vi "Z_state.vi"(9 "Alarm":bool[](array[boolean])=[FALSE, FALSE], 10 "Z_In":T4={"Z_Source"=enum."hand", "Z_Set_State"=enum."initialization", "ZM_State"=enum."initialization"}, 11 "HE1_Z_state in":refnum<class "HE_Z_state.lvclass">) -> (3 "HE1_Z_state out":refnum<class "HE_Z_state.lvclass">)   [LabVIEW 2019, in "Heating.lvlib" / "HE_Z_state.lvclass"]
uses:
  HE_Z_state.lvclass
  D:/my_projects/projects/Algorithms/Labview/19/Sequence/State/State.lvclass
  ctl/Z_source.ctl
  ctl/Z_State.ctl
  ctl/ZM_State.ctl
  HE_Z_state.lvclass/HE_Z_state.ctl
  Sequence/State/State.lvclass
  Heating.lvlib
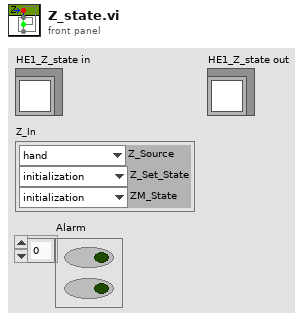
[diagram p1: front panel]
types:
  T1 = typedef "Heating.lvlib/Z_source.ctl" = enum8{"initialize", "local disabled", "local hand", "hand", "auto", "dist"}
  T2 = typedef "Heating.lvlib/Z_State.ctl" = enum8{"initialization", "alarm", "disabled", "not ready", "stop ready", "reserv", "switched off", "reserv2", "switched on", "check", "on min", "decrease out", "on", "increase out", "on max"}
  T3 = typedef "Heating.lvlib/ZM_State.ctl" = enum8{"initialization", "stop", "start_cmd", "contactor_on_cmd", "heating", "on", "stop_cmd", "power_down", "contactor_off_cmd", "cooling", "restart_delay"}
  T4 = cluster{"Z_Source":T1, "Z_Set_State":T2, "ZM_State":T3}
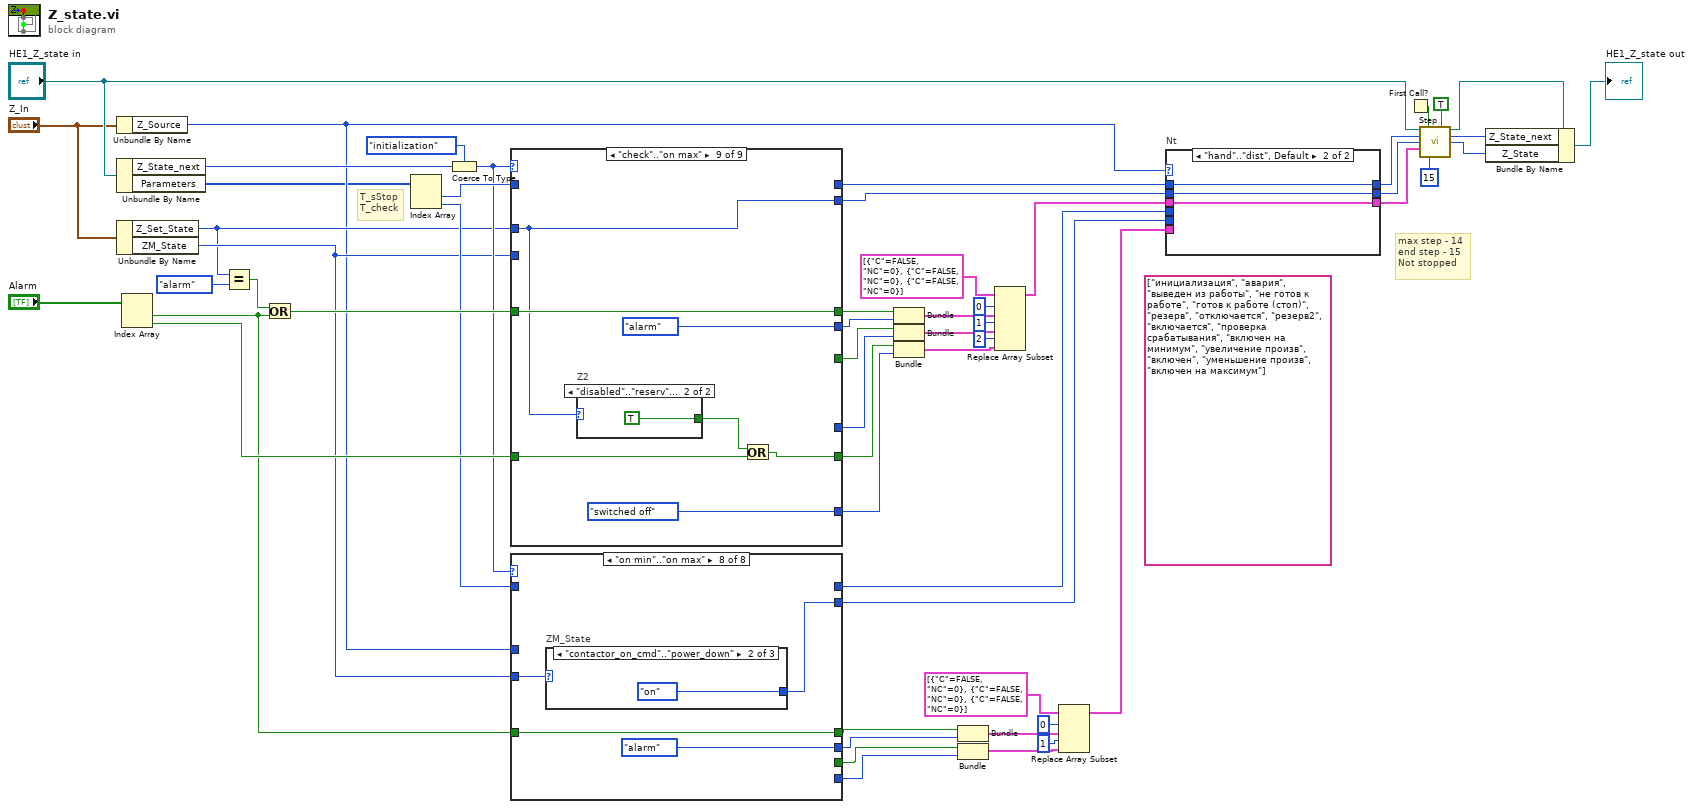
[diagram p0: block diagram]
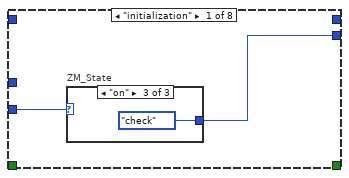
[diagram p2: hidden frame]
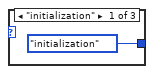
[diagram p3: hidden frame]
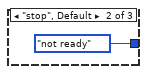
[diagram p4: hidden frame]
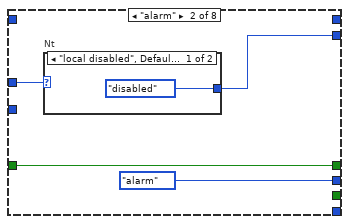
[diagram p5: hidden frame]
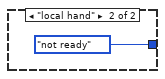
[diagram p6: hidden frame]
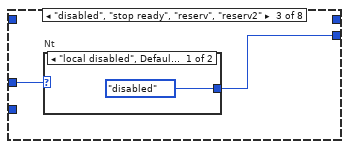
[diagram p7: hidden frame]
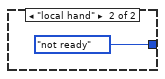
[diagram p8: hidden frame]
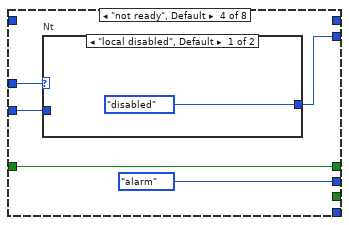
[diagram p9: hidden frame]
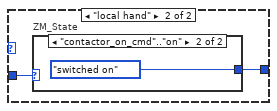
[diagram p10: hidden frame]
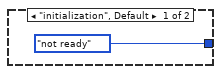
[diagram p11: hidden frame]
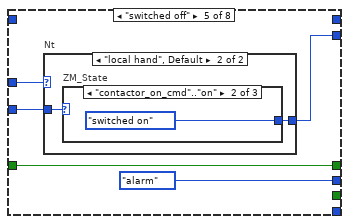
[diagram p12: hidden frame]
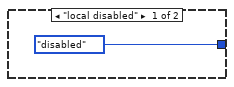
[diagram p13: hidden frame]
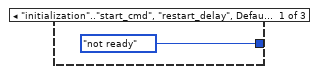
[diagram p14: hidden frame]
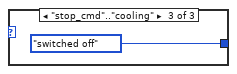
[diagram p15: hidden frame]
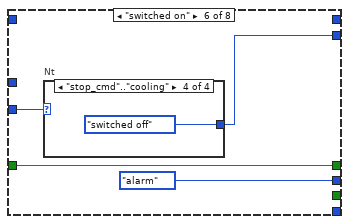
[diagram p16: hidden frame]
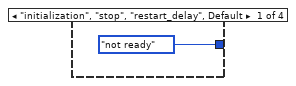
[diagram p17: hidden frame]
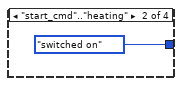
[diagram p18: hidden frame]
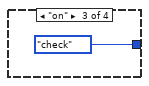
[diagram p19: hidden frame]
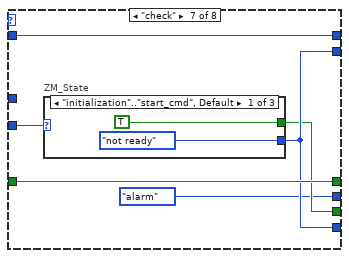
[diagram p20: hidden frame]
diagram:
  (unwired) string[] ["инициализация", "авария", "выведен из работы", "не готов к работе", "готов к работе (стоп)", "резерв", "отключается", "резерв2", "включается", "проверка срабатывания", "включен на минимум", "увеличение произв", "включен", "уменьшение произв", "включен на максимум"]
  # "T_sStop\nT_check"
  # "max step - 14\nend step - 15\nNot stopped"
  n1 = Unbundle By Name("Z_In") -> ("Z_Source"=w8:T1)
  n2 = Unbundle By Name("HE1_Z_state in") -> ("Z_State_next"=w9:T2, "Parameters"=w1:u32[])
  n3 = Unbundle By Name("Z_In") -> ("Z_Set_State"=w10:T2, "ZM_State"=w11:T3)
  n4 = Index Array(array="Alarm") -> (element #1=w17:bool, element #2=w39:bool)  [unwired: 2 in]
  n5 = Equal?(x=w10, y=Z_State."alarm") -> (x = y?=w44:bool)
  n6 = Or(x=w44, y=w17) -> (x .or. y?=w43:bool)
  n7 = Index Array(array=w1) -> (element #1=w40:u32, element #2=w19:u32)  [unwired: 2 in]
  n8 = Coerce To Type(0:w9, 1:Z_State."initialization" ("Z_SetState")) -> (2:w18:T2)
  n9 = case shown="\"check\"..\"on max\"" w18 {
    tunnel: w43 -> [_ w64 w71 w79 w89 w109 w121 w137 w152]
    tunnel: w10 -> [w56 w65 w72 w80 w93 w110 w122 w135 w148]
    tunnel: w39 -> [_ _ _ w77 w91 w108 w118 w138 w150]
    tunnel: w40 -> [_ _ _ _ w92 _ _ _ _]
    tunnel: w11 -> [w58 _ _ _ w94 _ w115 w141 _]
    tunnel: [_ _ _ Z_State."not ready" ("Z_SetState") Z_State."not ready" ("Z_SetState") Z_State."not ready" ("Z_SetState") w114 Z_State."switched off" ("Z_SetState") Z_State."switched off" ("Z_SetState")] -> w23
    tunnel: [_ _ _ _ w92 _ _ _ _] -> w2
    tunnel: [_ _ _ w77 w91 w108 w118 w140 w151] -> w22
    tunnel: [_ _ _ _ Z_State."disabled" ("Z_SetState") _ w119 _ _] -> w21
    tunnel: [_ _ _ _ w90 _ w120 _ _] -> w24
    tunnel: [_ Z_State."alarm" ("Z_SetState") Z_State."alarm" ("Z_SetState") Z_State."alarm" ("Z_SetState") Z_State."alarm" ("Z_SetState") Z_State."alarm" ("Z_SetState") Z_State."alarm" ("Z_SetState") Z_State."alarm" ("Z_SetState") Z_State."alarm" ("Z_SetState")] -> w25
    tunnel: [_ w64 w71 w79 w89 w109 w121 w137 w152] -> w26
    tunnel: [w57 w63 w70 w78 w88 w107 w117 w136 w148] -> w3
    frame "initialization" {
      n10 = case "ZM_State" shown="\"on\"" w58 {
        tunnel: [Z_State."initialization" ("Z_SetState") Z_State."not ready" ("Z_SetState") w61] -> w57
        tunnel: w56 -> [_ _ w61]
        frame "initialization" {
        }
        frame "stop", Default {
        }
        frame "on" {
        }
      }
    }
    frame "alarm" {
      n11 = case "Nt" shown="\"disabled\"" w65 {
        tunnel: [Z_State."alarm" ("Z_SetState") Z_State."disabled" ("Z_SetState") Z_State."not ready" ("Z_SetState")] -> w63
        frame "alarm", Default {
        }
        frame "disabled" {
        }
        frame "not ready".."on max" {
        }
      }
    }
    frame "disabled" {
      n12 = case "Nt" shown="\"not ready\"..\"on max\"" w72 {
        tunnel: [Z_State."disabled" ("Z_SetState") Z_State."not ready" ("Z_SetState")] -> w70
        frame "alarm", "disabled", Default {
        }
        frame "not ready".."on max" {
        }
      }
    }
    frame "not ready", Default {
      n13 = case "Nt" shown="\"disabled\"" w80 {
        tunnel: [Z_State."alarm" ("Z_SetState") Z_State."disabled" ("Z_SetState") Z_State."not ready" ("Z_SetState") Z_State."stop ready" ("Z_SetState")] -> w78
        frame "alarm", Default {
        }
        frame "disabled" {
        }
        frame "not ready" {
        }
        frame "stop ready".."on max" {
        }
      }
    }
    frame "stop ready" {
      n14 = case "Nt" shown="\"on min\"..\"on max\"" w93 {
        tunnel: [Z_State."stop ready" ("Z_SetState") w97 w101] -> w88
        tunnel: w94 -> [_ w98 w102]
        frame "stop ready", Default {
        }
        frame "reserv" {
          n15 = case "ZM_State" shown="\"initialization\", Default" w98 {
            tunnel: [Z_State."reserv" ("Z_SetState") Z_State."stop ready" ("Z_SetState")] -> w97
            frame "initialization", Default {
            }
            frame "restart_delay" {
            }
          }
        }
        frame "on min".."on max" {
          n16 = case "ZM_State" shown="\"initialization\", Default" w102 {
            tunnel: [Z_State."switched on" ("Z_SetState") Z_State."stop ready" ("Z_SetState")] -> w101
            frame "initialization", Default {
            }
            frame "restart_delay" {
            }
          }
        }
      }
      n17 = Equal?(x=w93, y=Z_State."disabled") -> (x = y?=w90:bool)
    }
    frame "reserv" {
      n18 = case "Nt" shown="\"check\"..\"on max\"" w110 {
        selector: w110 -> [w111 _ _]
        tunnel: [w111 Z_State."stop ready" ("Z_SetState") Z_State."switched on" ("Z_SetState")] -> w107
        frame "alarm".."not ready", "reserv" {
        }
        frame "stop ready", Default {
        }
        frame "check".."on max" {
        }
      }
    }
    frame "switched off" {
      n19 = case "Nt" shown="\"stop ready\", \"reserv\", \"check\", Default" w122 {
        tunnel: [w128 Z_State."switched on" ("Z_SetState")] -> w117
        tunnel: w115 -> [w129 _]
        frame "stop ready", "reserv", "check", Default {
          n20 = case "ZM_State" shown="\"on\"..\"cooling\"" w129 {
            tunnel: [Z_State."stop ready" ("Z_SetState") Z_State."switched off" ("Z_SetState")] -> w128
            frame "initialization", Default {
            }
            frame "on".."cooling" {
            }
          }
        }
        frame "on min".."on max" {
        }
      }
      n21 = case "ZM_State" shown="\"on\"..\"cooling\"" w115 {
        tunnel: [Z_State."disabled" ("Z_SetState") Z_State."switched off" ("Z_SetState")] -> w119
        frame "initialization", "stop", "restart_delay", Default {
        }
        frame "on".."cooling" {
        }
      }
      n22 = case "ZM_State" shown="\"on\"..\"cooling\"" w115 {
        tunnel: [Z_State."not ready" ("Z_SetState") Z_State."switched off" ("Z_SetState")] -> w114
        frame "initialization", "stop", "restart_delay", Default {
        }
        frame "on".."cooling" {
        }
      }
      n23 = Equal?(x=w122, y=Z_State."disabled") -> (x = y?=w120:bool)
    }
    frame "switched on" {
      n24 = case "ZM_State" shown="\"initialization\", Default" w141 {
        tunnel: [Z_State."switched on" ("Z_SetState") w143] -> w136
        tunnel: w135 -> [_ w143]
        frame "initialization", Default {
        }
        frame "on" {
        }
      }
      n25 = case "Z2" shown="\"disabled\"..\"reserv\", Default" w135 {
        tunnel: [FALSE TRUE] -> w139
        frame "check".."on max" {
        }
        frame "disabled".."reserv", Default {
        }
      }
      n26 = Or(x=w139, y=w138) -> (x .or. y?=w140:bool)
    }
    frame "check".."on max" {
      n27 = case "Z2" shown="\"disabled\"..\"reserv\", Default" w148 {
        tunnel: [FALSE TRUE] -> w149
        frame "check".."on max" {
        }
        frame "disabled".."reserv", Default {
        }
      }
      n28 = Or(x=w149, y=w150) -> (x .or. y?=w151:bool)
    }
  }
  n29 = case shown="\"on min\"..\"on max\"" w18 {
    tunnel: w17 -> [_ w163 _ w174 w184 w194 w204 w214]
    tunnel: w8 -> [_ w162 w167 w173 w183 _ _ _]
    tunnel: w11 -> [w156 _ _ w171 w182 w193 w203 w212]
    tunnel: [_ _ _ _ _ _ w202 _] -> w13
    tunnel: [_ _ _ _ _ _ w201 _] -> w14
    tunnel: [_ Z_State."alarm" ("Z_SetState") _ Z_State."alarm" ("Z_SetState") Z_State."alarm" ("Z_SetState") Z_State."alarm" ("Z_SetState") Z_State."alarm" ("Z_SetState") Z_State."alarm" ("Z_SetState")] -> w15
    tunnel: [_ w163 _ w174 w184 w194 w204 w214] -> w16
    tunnel: [w155 w161 w166 w172 w181 w192 w202 w211] -> w4
    tunnel: w19 -> [_ _ _ _ _ _ w200 _]
    tunnel: [_ _ _ _ _ _ w200 _] -> w5
    frame "initialization" {
      n30 = case "ZM_State" shown="\"on\"" w156 {
        tunnel: [Z_State."initialization" ("Z_SetState") Z_State."not ready" ("Z_SetState") Z_State."check" ("Z_SetState")] -> w155
        frame "initialization" {
        }
        frame "stop", Default {
        }
        frame "on" {
        }
      }
    }
    frame "alarm" {
      n31 = case "Nt" shown="\"local disabled\", Default" w162 {
        tunnel: [Z_State."disabled" ("Z_SetState") Z_State."not ready" ("Z_SetState")] -> w161
        frame "local disabled", Default {
        }
        frame "local hand" {
        }
      }
    }
    frame "disabled", "stop ready", "reserv", "reserv2" {
      n32 = case "Nt" shown="\"local disabled\", Default" w167 {
        tunnel: [Z_State."disabled" ("Z_SetState") Z_State."not ready" ("Z_SetState")] -> w166
        frame "local disabled", Default {
        }
        frame "local hand" {
        }
      }
    }
    frame "not ready", Default {
      n33 = case "Nt" shown="\"local disabled\", Default" w173 {
        tunnel: [Z_State."disabled" ("Z_SetState") w177] -> w172
        tunnel: w171 -> [_ w176]
        frame "local disabled", Default {
        }
        frame "local hand" {
          n34 = case "ZM_State" shown="\"contactor_on_cmd\"..\"on\"" w176 {
            tunnel: [Z_State."not ready" ("Z_SetState") Z_State."switched on" ("Z_SetState")] -> w177
            frame "initialization", Default {
            }
            frame "contactor_on_cmd".."on" {
            }
          }
        }
      }
    }
    frame "switched off" {
      n35 = case "Nt" shown="\"local hand\", Default" w183 {
        tunnel: [Z_State."disabled" ("Z_SetState") w186] -> w181
        tunnel: w182 -> [_ w187]
        frame "local disabled" {
        }
        frame "local hand", Default {
          n36 = case "ZM_State" shown="\"contactor_on_cmd\"..\"on\"" w187 {
            tunnel: [Z_State."not ready" ("Z_SetState") Z_State."switched on" ("Z_SetState") Z_State."switched off" ("Z_SetState")] -> w186
            frame "initialization".."start_cmd", "restart_delay", Default {
            }
            frame "contactor_on_cmd".."on" {
            }
            frame "stop_cmd".."cooling" {
            }
          }
        }
      }
    }
    frame "switched on" {
      n37 = case "Nt" shown="\"stop_cmd\"..\"cooling\"" w193 {
        tunnel: [Z_State."not ready" ("Z_SetState") Z_State."switched on" ("Z_SetState") Z_State."check" ("Z_SetState") Z_State."switched off" ("Z_SetState")] -> w192
        frame "initialization", "stop", "restart_delay", Default {
        }
        frame "start_cmd".."heating" {
        }
        frame "on" {
        }
        frame "stop_cmd".."cooling" {
        }
      }
    }
    frame "check" {
      n38 = case "ZM_State" shown="\"initialization\"..\"start_cmd\", Default" w203 {
        tunnel: [Z_State."not ready" ("Z_SetState") Z_State."on" ("Z_SetState") Z_State."switched off" ("Z_SetState")] -> w202
        tunnel: [TRUE FALSE TRUE] -> w201
        frame "initialization".."start_cmd", Default {
        }
        frame "contactor_on_cmd".."power_down" {
        }
        frame "contactor_off_cmd".."restart_delay" {
        }
      }
    }
    frame "on min".."on max" {
      n39 = case "ZM_State" shown="\"contactor_on_cmd\"..\"power_down\"" w212 {
        tunnel: [Z_State."not ready" ("Z_SetState") Z_State."on" ("Z_SetState") Z_State."switched off" ("Z_SetState")] -> w211
        frame "initialization".."start_cmd", Default {
        }
        frame "contactor_on_cmd".."power_down" {
        }
        frame "contactor_off_cmd".."restart_delay" {
        }
      }
    }
  }
  n40 = Bundle(w26, "Z_SetState"=w25) -> (w36:cluster{bool, "Z_SetState":T2})  [unwired: 1 in]
  n41 = Bundle(w24, "Z_SetState"=w21) -> (w33:cluster{bool, "Z_SetState":T2})  [unwired: 1 in]
  n42 = Bundle("Alarm"=w22, "Z_SetState"=w23) -> (w32:cluster{"Alarm":bool, "Z_SetState":T2})  [unwired: 1 in]
  n43 = Bundle("Alarm"=w16, "Z_SetState"=w15) -> (w29:cluster{"Alarm":bool, "Z_SetState":T2})  [unwired: 1 in]
  n44 = Bundle(w14, "Z_SetState"=w13) -> (w31:cluster{bool, "Z_SetState":T2})  [unwired: 1 in]
  n45 = Replace Array Subset(array=cluster{"C":bool, "NC":u32}[] [{"C"=FALSE, "NC"=0}, {"C"=FALSE, "NC"=0}, {"C"=FALSE, "NC"=0}] ("appended array"), new element #1=w36, index #1=0 ("index"), new element #2=w33, index #2=1 ("index"), new element #3=w32, index #3=2 ("index")) -> (w6:cluster{"C":bool, "NC":u32}[])
  n46 = Replace Array Subset(array=cluster{"C":bool, "NC":u32}[] [{"C"=FALSE, "NC"=0}, {"C"=FALSE, "NC"=0}, {"C"=FALSE, "NC"=0}] ("appended array"), new element #1=w29, index #1=0 ("index"), new element #2=w31, index #2=1 ("index")) -> (w7:cluster{"C":bool, "NC":u32}[])
  n47 = case "Nt" shown="\"hand\"..\"dist\", Default" w8 {
    tunnel: w3 -> [_ w223]
    tunnel: w6 -> [_ w222]
    tunnel: [w219 w223] -> w50
    tunnel: [w220 w222] -> w51
    tunnel: w4 -> [w219 _]
    tunnel: w7 -> [w220 _]
    tunnel: w2 -> [_ w221]
    tunnel: [w218 w221] -> w49
    tunnel: w5 -> [w218 _]
    frame "local disabled", "local hand" {
    }
    frame "hand".."dist", Default {
    }
  }
  n48 = First Call?() -> (First Call?: T/F=w55:bool)
  n49 = call "Step.vi"("State in"="HE1_Z_state in", "Reset"=w55, "Start in"=TRUE ("Start"), "t"=w49, "Nt"=w50, "C_table"=w51, "N end step"=u32 15) -> ("State out"=w45:refnum<class "HE_Z_state.lvclass">, "N next"=w52:u32, "N curr"=w53:u32)  [unwired: 5 in, 1 out]
  n50 = Bundle By Name(cluster=w45, "Z_State_next"=w52, "Z_State"=w53) -> (→"HE1_Z_state out":refnum<class "HE_Z_state.lvclass">)
